vi "toString.vi"(7 "UTC? (F)":bool, 9 "Timestamp (now)":timestamp, 11 "DateTimeFormatter in":refnum<class "DateTimeFormatter.lvclass">) -> (1 "DateTime String":string, 3 "DateTimeFormatter out":refnum<class "DateTimeFormatter.lvclass">)   [LabVIEW 2013, in "DateTimeFormatter.lvclass"]
uses:
  DateTimeFormatter.lvclass
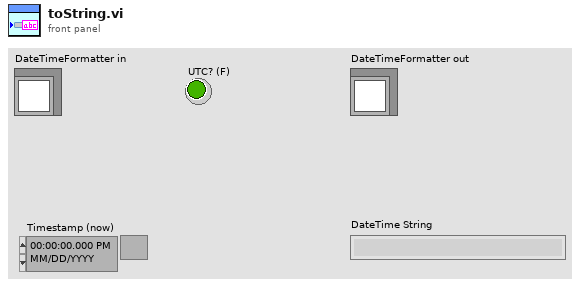
[diagram p1: front panel]
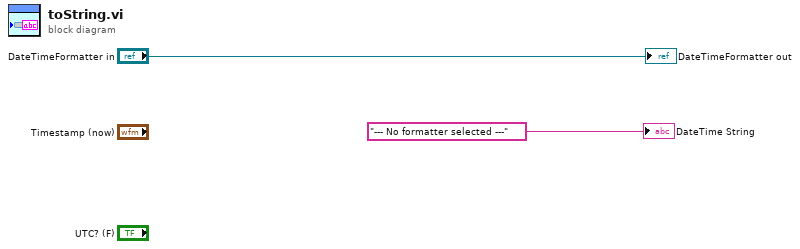
[diagram p0: block diagram]
diagram:
  "DateTimeFormatter out" <- "DateTimeFormatter in"
  "DateTime String" <- "--- No formatter selected ---" ("DateTime String")
